vi "ExPickStrip.vi"() -> ()   [LabVIEW 2010]
panel:
  in  "Trigger Edge":u32(ring)=1 items=["", "Positive (leading) edge", "Negative (falling) Edge"]
  in  "Trigger/Timing Mode":u32(ring)=1 items=["N/A", "FreeRun/Timed", "Single Trigger (PM only)", "Ext Sync/Strobed", "Bulb (PM only)", "Variable (PM only)", "Flash Mode (PM only)"]
  in  "Strip":u32=1 min=1 step=1
  out "Strip":sgl[](graph)
  in  "Temperature":dbl=-10.0 format="%.2f"
  in  "Exposure":dbl min=0.0 step=0.001 format="%.3f"
  in  "stop":bool
  out "error out":errorcluster
  in  "error in (no error)":errorcluster
  # "ExPickStrip:\nThis example allows a strip to be picked before running. \nIt will then program up the strip and display it on the graph.\nNote: This example uses circular buffers, so camera must\nsupport circular buffers."
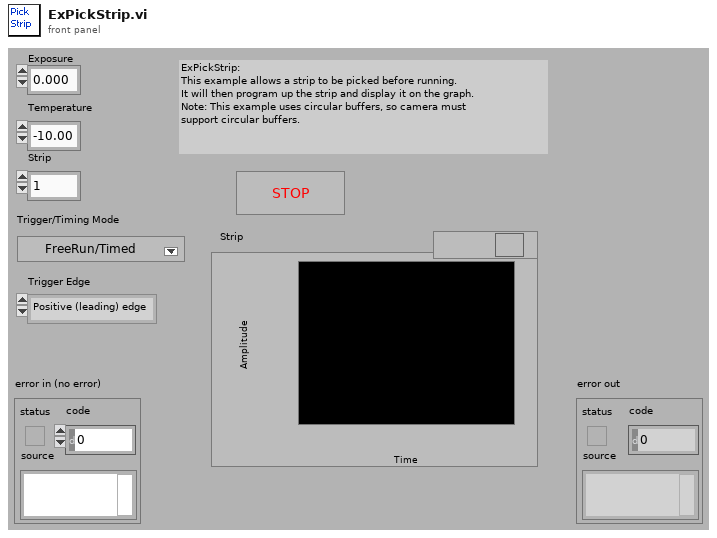
[diagram p1: front panel]
types:
  T1 = cluster{"Acquire Mode \n(1-Focus sync)\nNote: not all \ncamera support \nthis mode.":i32, "Exposure":dbl, "Number of frames":i32, "Software Accumulations":i32}
  T2 = cluster{"Camera Handle":u32, "Pulser Handle":u32, "File Handle":u32, "Display Handle":u32, "Image Handle":u32}
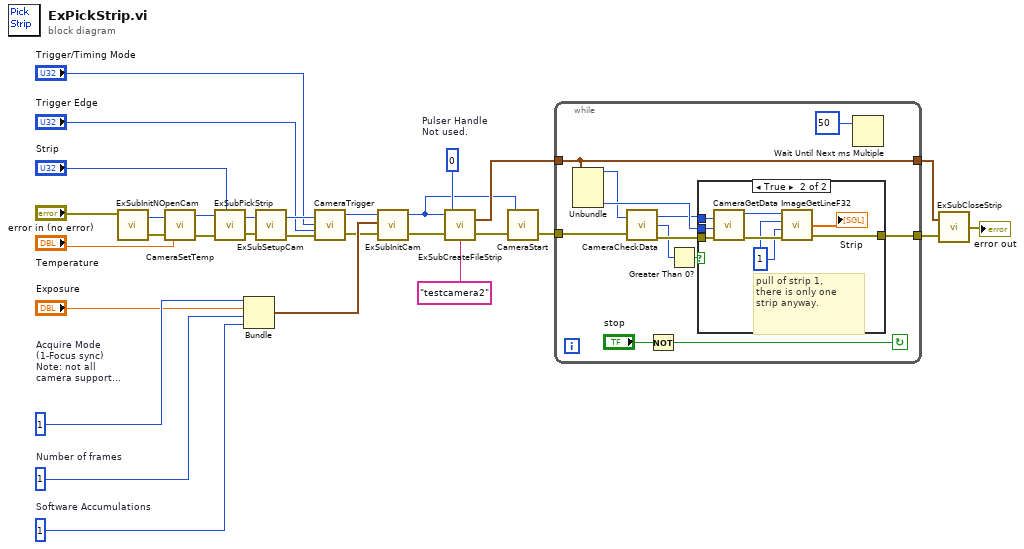
[diagram p0: block diagram]
diagram:
  w22 = 0  # Pulser Handle Not used.
  w28 = 1  # Number of frames
  w29 = 1  # Acquire Mode  (1-Focus sync) Note: not all  camera support  this mode.
  w27 = 1  # Software Accumulations
  n1 = call "ExSubInitNOpenCam.vi"("error in (no error)"="error in (no error)") -> ("Camera Handle"=w8:u32, "error out"=w9:errorcluster)
  n2 = call <userlib>:"CameraSetTemp.vi"("error in (no error)"=w9, "Temperature"="Temperature", "Camera Handle"=w8) -> ("error out"=w7:errorcluster, "Camera Handle"=w6:u32)
  n3 = call "ExSubPickStrip.vi"("error in (no error)"=w7, "Strip to display"="Strip", "Camera Handle"=w6) -> ("error out"=w4:errorcluster, "Camera Handle"=w3:u32)
  n4 = Bundle("Acquire Mode \n(1-Focus sync)\nNote: not all \ncamera support \nthis mode."=w29, "Exposure"="Exposure", "Number of frames"=w28, "Software Accumulations"=w27) -> (w24:T1)  [unwired: 1 in]
  n5 = call "ExSubSetupCam.vi"("error in (no error)"=w4, "Camera Handle"=w3) -> ("error out"=w13:errorcluster, "Camera Handle"=w15:u32)
  n6 = call <userlib>:"CameraTrigger.vi"("error in"=w13, "Trigger Edge"="Trigger Edge", "Timing Mode"="Trigger/Timing Mode", "Camera Handle"=w15) -> ("error out"=w16:errorcluster, "Camera Handle"=w14:u32)
  n7 = call "ExSubInitCam.vi"("error in (no error)"=w16, "Camera Information"=w24, "Camera Handle"=w14) -> ("error out"=w23:errorcluster, "Camera Handle"=w20:u32)
  n8 = call "ExSubCreateFileStrip.vi"("error in (no error)"=w23, "File and Display Name"="testcamera2", "Pulser Handle"=w22, "Camera Handle"=w20) -> ("error out"=w11:errorcluster, "Handles Out"=w21:T2)
  n9 = call <userlib>:"CameraStart.vi"("error in"=w11, "Camera Handle"=w20) -> ("error out"=w12:errorcluster)  [unwired: 1 out]
  n10 = while {
    tunnel: w21 -> [w39]
    tunnel: w12 -> [w38]
    tunnel: [w36] -> w18
    tunnel: [w39] -> w19
    stop <- w40 continue-if-true
    n11 = Unbundle(w39) -> ("Camera Handle"=w34:u32, "Image Handle"=w35:u32)  [unwired: 3 out]
    n12 = call <userlib>:"CameraCheckData.vi"("Camera Handle"=w34, "error in"=w38) -> ("Camera Handle"=w33:u32, "Number Of Frames Available"=w31:i32, "error out"=w37:errorcluster)
    n13 = Not(x="stop") -> (.not. x?=w40:bool)
    n14 = Greater Than 0?(x=w31) -> (x > 0?=w32:bool)
    n15 = case shown="True" w32 {
      tunnel: w37 -> [w43 w50]
      tunnel: [w43 w48] -> w36
      tunnel: w35 -> [_ w45]
      tunnel: w33 -> [_ w44]
      frame False {
      }
      frame True {
        w46 = 1
        # "pull of strip 1,\nthere is only one\nstrip anyway."
        n16 = call <userlib>:"CameraGetData.vi"("error in"=w50, "Data Handle"=w45, "Camera Handle"=w44) -> ("error out"=w49:errorcluster, "Data Handle"=w47:u32)  [unwired: 1 out]
        n17 = call <userlib>:"ImageGetLineF32.vi"("error in"=w49, "Z Position"=w46, "Y Position"=w46, "Data Handle"=w47) -> ("error out"=w48:errorcluster, "Array F32"=→"Strip":sgl[])  [unwired: 1 out]
      }
    }
    n18 = Wait Until Next ms Multiple(millisecond multiple=50) -> ()  [unwired: 1 out]
  }
  n19 = call "ExSubCloseStrip.vi"("error in (no error)"=w18, "Handles In"=w19) -> ("error out"=→"error out":errorcluster)
